vi "test_example_dll.vi"(8 "error in (no error)":errorcluster, 11 "number in":i32) -> (0 "error out":errorcluster, 3 "number out":i32)   [LabVIEW 2014]
doc: "Using generated dll to test it, using call dll."
uses:
  build/example_dll.dll
panel:
  in  "number in 2":i32
  out "square":i32
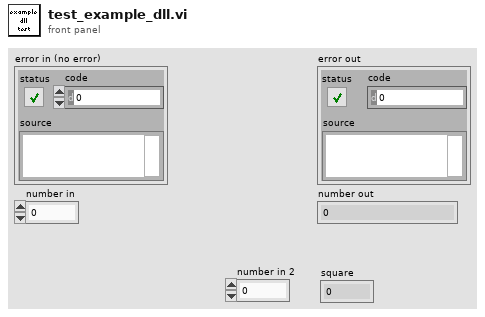
[diagram p1: front panel]
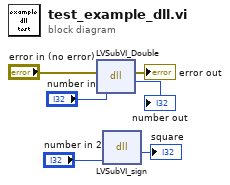
[diagram p0: block diagram]
diagram:
  n1 = dll-call lib="C:/Users/Simon Gurfunkel/Documents/LabVIEW_projects/LabVIEW-Transcript-DLL-Library/examples/1/build/example_dll.dll" fn="LVSubVI_Double"(error in="error in (no error)", "number in"="number in") -> (error out=→"error out":errorcluster, "number out"=→"number out":i32)  [unwired: 3 in, 1 out]
  n2 = dll-call lib="C:/Users/Simon Gurfunkel/Documents/LabVIEW_projects/LabVIEW-Transcript-DLL-Library/examples/1/build/example_dll.dll" fn="LVSubVI_sign"("number in"="number in 2") -> ("number out"=→"square":i32)  [unwired: 4 in, 2 out]
